vi "Scale Selector Test.vi"() -> ()   [LabVIEW 2015]
uses:
  Scale Selector/Scale Selector.xctl
panel:
  in  "Scale Selector":dbl(xcontrol)
  in  "stop":bool
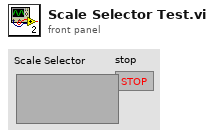
[diagram p1: front panel]
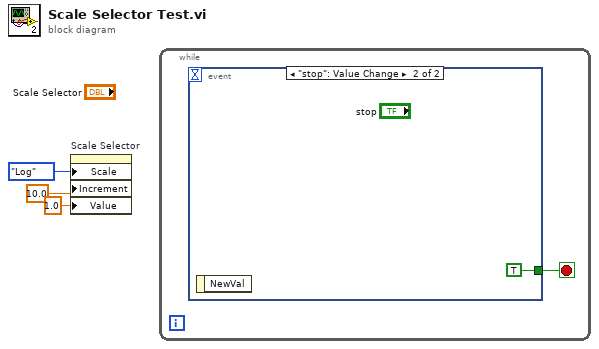
[diagram p0: block diagram]
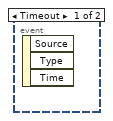
[diagram p2: hidden frame]
diagram:
  n1 = property on="Scale Selector" class="Scale Selector (strict)"("Scale"=enum16{"Linear", "Log"}."Log", "Increment"=10.0, "Value"=1.0 ("Scale Selector")) -> ()  [unwired: 2 in, 2 out]
  n2 = while {
    stop <- w4 stop-if-true
    n3 = event shown="[1] \"stop\": Value Change" {
      selector: _ -> [_ _]
      dyn-events: _ -> [_ _]
      timeout: _ -> [_ _]
      tunnel: [_ TRUE] -> w4
      event Timeout {
        n4 = event-data() -> ()  [unwired: 1 in, 3 out]
      }
      event "stop": Value Change {
        n5 = event-data() -> ()  [unwired: 1 in, 1 out]
      }
    }
  }
